vi "CAN MIL CEL Input FGV.vi"(8 "error in (no error)":errorcluster, 10 "CAN Input Channels":dbl[](array[numeric]), 11 "Action":enum16{"Set", "Get"}(ring)) -> (0 "error out":errorcluster, 2 "CAN Input Channels":dbl[](array[numeric]))   [LabVIEW 2018]
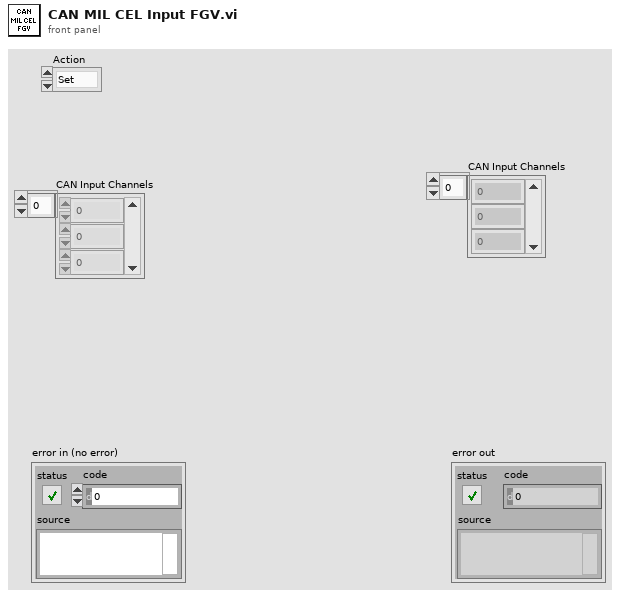
[diagram p1: front panel]
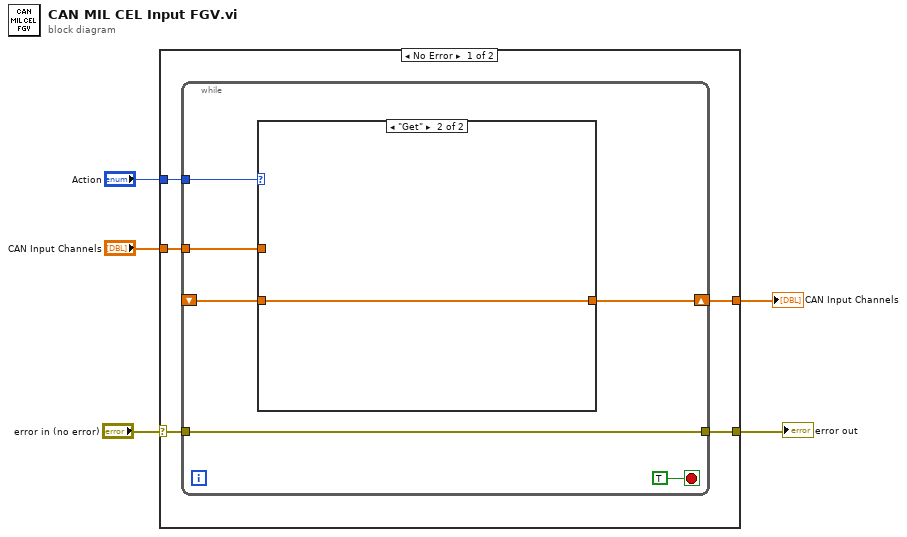
[diagram p0: block diagram]
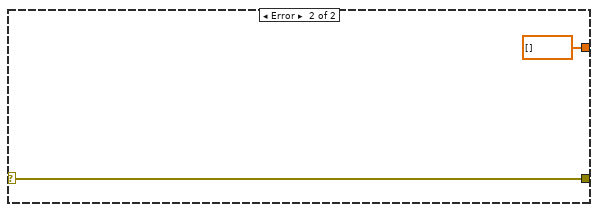
[diagram p3: hidden frame]
diagram:
  n1 = case shown="No Error" "error in (no error)" {
    selector: "error in (no error)" -> [w9 w20]
    tunnel: "Action" -> [w10 _]
    tunnel: [w8 w20] -> w3
    tunnel: "CAN Input Channels" -> [w7 _]
    tunnel: [w6 dbl[] [] ("PWM Input Channels")] -> w1
    frame No Error {
      n2 = while {
        tunnel: w10 -> [w16]
        tunnel: [w14] -> w8
        tunnel: w9 -> [w14]
        tunnel: w7 -> [w13]
        shift-right: [w12] -> w6
        shift-left: _ -> [w11]
        stop <- TRUE stop-if-true
        n3 = case shown="\"Get\"" w16 {
          tunnel: w13 -> [w17 _]
          tunnel: [w17 w18] -> w12
          tunnel: w11 -> [_ w18]
          frame "Set", Default {
          }
          frame "Get" {
          }
        }
      }
    }
    frame Error {
    }
  }
  "error out" <- w3
  "CAN Input Channels" <- w1
